vi "WSVCAP SHL Host TL I2C Read.vi"(0 "Bytes to Read":u8=8, 5 "Sub Address [U8]":u8=191 format="%.0x", 7 "Socket Mask Set [U64]":u64[](array[numeric]) format="%012x", 11 "error in":errorcluster, 13 "Log (T)":bool=TRUE, 14 "FPGA":T1) -> (4 "C1 Read Data Out":u8[][](array[numeric]) format="%.0x", 6 "C2 Read Data Out":u8[][](array[numeric]) format="%.0x", 8 "C3 Read Data Out":u8[][](array[numeric]) format="%.0x", 15 "error out":errorcluster)   [LabVIEW 2012]
uses:
  Type Defs/WSVCAP SHL I2C FPGA Enum.ctl
  Type Defs/WSVCAP SHL Function Enum.ctl
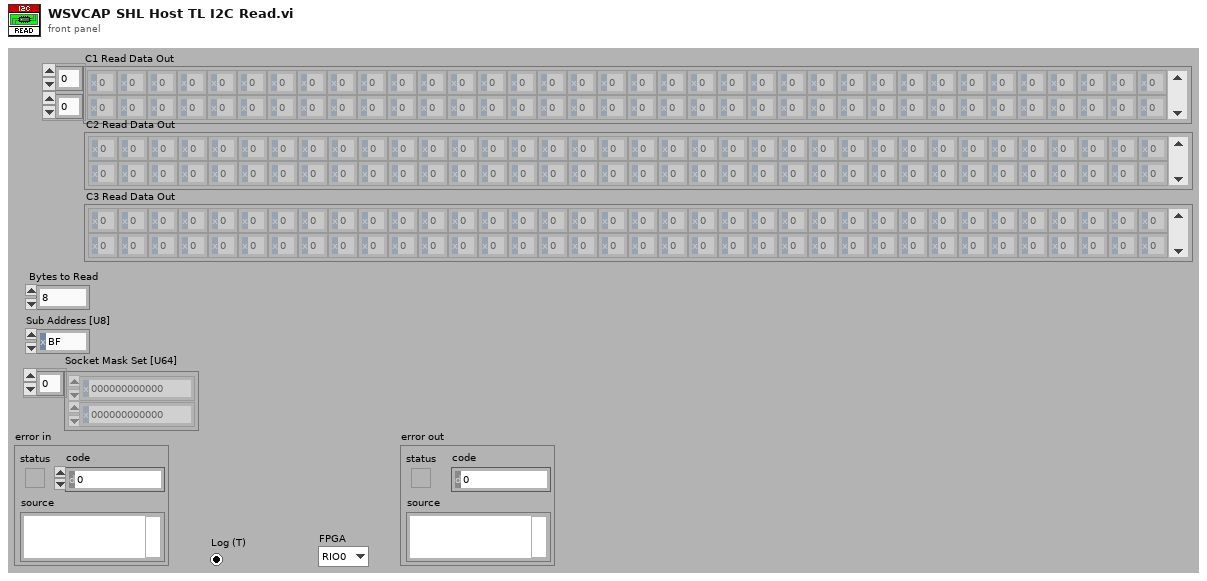
[diagram p1: front panel]
types:
  T1 = typedef "WSVCAP SHL I2C FPGA Enum.ctl" = enum16{"RIO0", "RIO1"}
  T2 = typedef "WSVCAP SHL Function Enum.ctl" = enum16{"Initialize", "Configure I2C", "Configure RFFE", "Write I2C", "Read I2C", "Write RFFE", "Read RFFE", "Start RFFE Cycle", "Stop RFFE Cycle", "Get Status", "Close"}
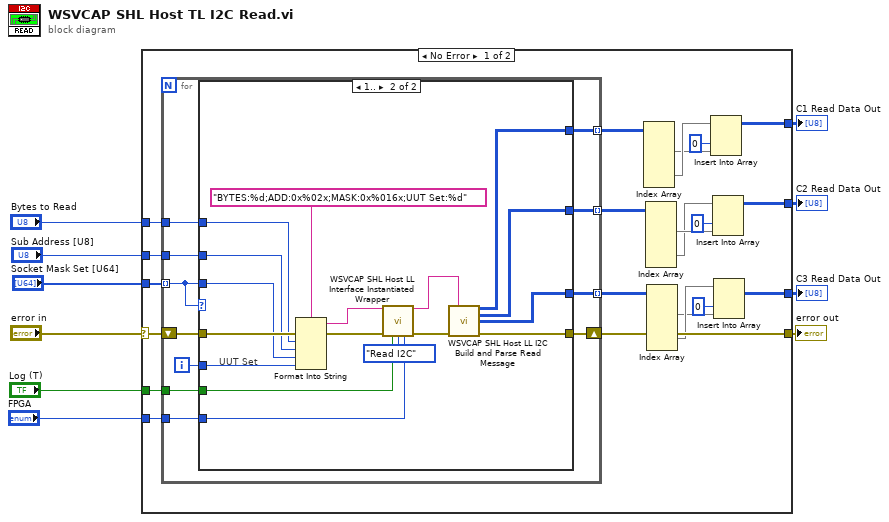
[diagram p0: block diagram]
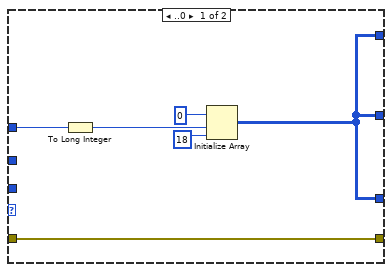
[diagram p2: hidden frame]
diagram:
  n1 = case shown="No Error" "error in" {
    selector: "error in" -> [w31 w67]
    tunnel: [w32 w67] -> w9
    tunnel: [w23 _] -> w4
    tunnel: [w14 _] -> w3
    tunnel: "Bytes to Read" -> [w30 _]
    tunnel: "Sub Address [U8]" -> [w29 _]
    tunnel: "Socket Mask Set [U64]" -> [w28 _]
    tunnel: "Log (T)" -> [w27 _]
    tunnel: [w12 _] -> w2
    tunnel: "FPGA" -> [w11 _]
    frame No Error {
      n2 = for {
        tunnel: [w42] -> w15 mode=indexing
        tunnel: w30 -> [w40]
        tunnel: w29 -> [w39]
        tunnel: w28 -> [w36] mode=indexing
        tunnel: w27 -> [w38]
        tunnel: [w37] -> w13 mode=indexing
        tunnel: [w35] -> w22 mode=indexing
        shift-right: [w43] -> w32
        shift-left: w31 -> [w41]
        tunnel: w11 -> [w33]
        i -> [w34]
        n3 = case shown="1.." w36 {
          tunnel: [w49 w65] -> w43
          tunnel: [w45 w63] -> w35
          tunnel: [w45 w62] -> w42
          tunnel: w41 -> [w49 w61]
          tunnel: w40 -> [w46 w58]
          tunnel: w39 -> [_ w57]
          tunnel: w36 -> [_ w56]
          tunnel: w38 -> [_ w53]
          tunnel: [w45 w52] -> w37
          tunnel: w34 -> [_ w51]
          tunnel: w33 -> [_ w50]
          frame ..0 {
            n4 = To Long Integer(number=w46) -> (32bit integer=w44:i32)
            n5 = Initialize Array(u8 0 ("Read Data"), w44, 18 ("Read Data")) -> (w45:u8[][])
          }
          frame 1.. {
            # "UUT Set"
            n6 = Format Into String(format string="BYTES:%d;ADD:0x%02x;MASK:0x%016x;UUT Set:%d", error in=w61, w58, w57, w56, w51) -> (resulting string=w55:string, error out=w60:errorcluster)  [unwired: 1 in]
            n7 = call "WSVCAP SHL Host LL Interface Instantiated Wrapper.vi"("Message In"=w55, "error in"=w60, "Log (T)"=w53, "Function"=WSVCAP_SHL_Function_Enum."Read I2C", "FPGA"=w50) -> ("Message Out"=w64:string, "error out"=w66:errorcluster)  [unwired: 8 in, 1 out]
            n8 = call "WSVCAP SHL Host LL I2C Build and Parse Read Message.vi"("Message In"=w64, "error in"=w66) -> ("C1 Read Data Out"=w63:u8[][], "C2 Read Data Out"=w62:u8[][], "C3 Read Data Out"=w52:u8[][], "error out"=w65:errorcluster)  [unwired: 8 in, 2 out]
          }
        }
      }
      n9 = Index Array(array=w22) -> (element #1=w25:u8[][], element #2=w26:u8[][])  [unwired: 6 in]
      n10 = Index Array(array=w15) -> (element #1=w20:u8[][], element #2=w19:u8[][])  [unwired: 6 in]
      n11 = Index Array(array=w13) -> (element #1=w17:u8[][], element #2=w18:u8[][])  [unwired: 6 in]
      n12 = Insert Into Array(array=w26, index (col)=0 ("disabled index (col)"), new element=w25) -> (w23:u8[][])  [unwired: 1 in]
      n13 = Insert Into Array(array=w19, index (col)=0 ("disabled index (col)"), new element=w20) -> (w14:u8[][])  [unwired: 1 in]
      n14 = Insert Into Array(array=w18, index (col)=0 ("disabled index (col)"), new element=w17) -> (w12:u8[][])  [unwired: 1 in]
    }
    frame Error {
    }
  }
  "error out" <- w9
  "C3 Read Data Out" <- w2
  "C1 Read Data Out" <- w4
  "C2 Read Data Out" <- w3
